vi "fgv_vlp16_enable.vi"(7 "cmd":enum16{"init", "read", "write"}(ring)=enum."write", 11 "v range":cluster{i8, i8}(slide)={15, -15} scale=-15.0..15.0) -> (3 "Enable vlp ch out":bool[](array[boolean])=[TRUE, TRUE, TRUE, TRUE, TRUE, TRUE, TRUE, TRUE, TRUE, TRUE, TRUE, TRUE, TRUE, TRUE, TRUE, TRUE])   [LabVIEW 2019]
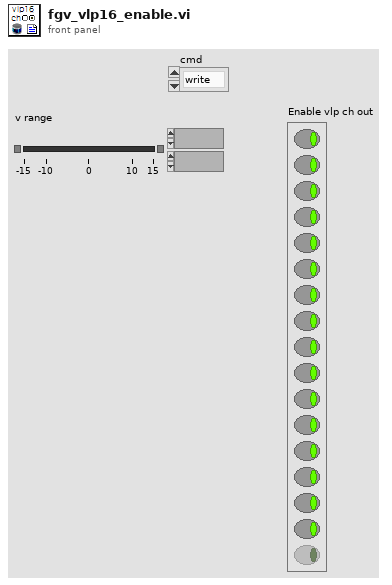
[diagram p1: front panel]
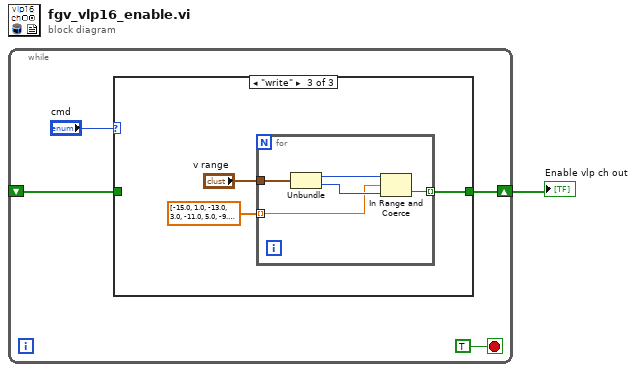
[diagram p0: block diagram]
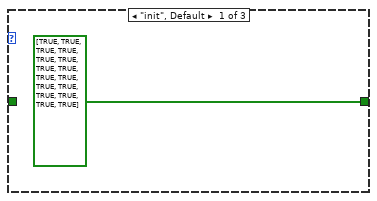
[diagram p2: hidden frame]
diagram:
  n1 = while {
    shift-right: [w3] -> w1
    shift-left: _ -> [w2]
    stop <- TRUE stop-if-true
    n2 = case shown="\"write\"" "cmd" {
      tunnel: [bool[] [TRUE, TRUE, TRUE, TRUE, TRUE, TRUE, TRUE, TRUE, TRUE, TRUE, TRUE, TRUE, TRUE, TRUE, TRUE, TRUE] ("Enable vlp ch") w7 w8] -> w3
      tunnel: w2 -> [_ w7 _]
      frame "init", Default {
      }
      frame "read" {
      }
      frame "write" {
        n3 = for {
          tunnel: dbl[] [-15.0, 1.0, -13.0, 3.0, -11.0, 5.0, -9.0, 7.0, -7.0, 9.0, -5.0, 11.0, -3.0, 13.0, -1.0, 15.0] -> [w13] mode=indexing
          tunnel: [w12] -> w8 mode=indexing
          tunnel: "v range" -> [w11]
          n4 = Unbundle(w11) -> (w15:i8, w14:i8)
          n5 = In Range and Coerce(upper limit=w15, x=w13, lower limit=w14) -> (In Range?=w12:bool)  [unwired: 1 out]
        }
      }
    }
  }
  "Enable vlp ch out" <- w1
